vi "ReferenceMove Core.vi"(8 "error in (no error)":errorcluster, 10 "AxisNumber":u8, 11 "CS++Nanotec in":refnum<class "CS++Nanotec.lvclass">) -> (0 "error out":errorcluster, 3 "CS++Nanotec out":refnum<class "CS++Nanotec.lvclass">)   [LabVIEW 2015, in "CS++Nanotec.lvlib" / "CS++Nanotec.lvclass"]
doc: "Starts a movement to the reference switch of this axis. Once the motor reaches the reference switch it should slowly move down from the switch and stop. Afterwards the internal step counter is set to zero. \n\nThe main purpose of this function is to calibrate the motor."
uses:
  CS++Nanotec.lvclass
  CS++Nanotec.lvclass/CS++Nanotec.ctl
  instr.lib/NanotecSMCPD/NanotecSMCPDDriver.lvlib
  CSPP_DeviceBase/CS++Motor/CS++Motor.lvclass
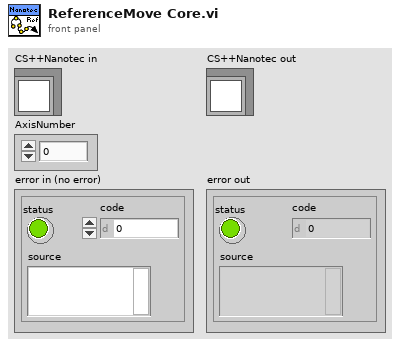
[diagram p1: front panel]
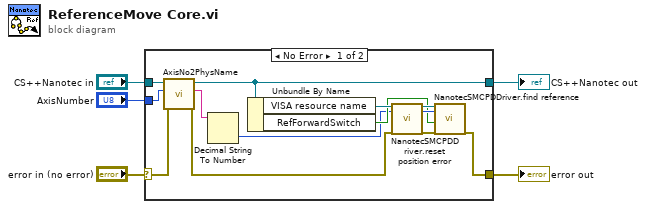
[diagram p0: block diagram]
diagram:
  n1 = case shown="No Error" "error in (no error)" {
    selector: "error in (no error)" -> [w9 w19]
    tunnel: "CS++Nanotec in" -> [w11 w20]
    tunnel: [w18 w19] -> w3
    tunnel: "AxisNumber" -> [w7 _]
    tunnel: [w10 w20] -> w1
    frame No Error {
      n2 = call "AxisNo2PhysName.vi"("error in (no error)"=w9, "AxisNumber"=w7, "CS++Motor in"=w11) -> ("error out"=w8:errorcluster, "PhysicalChannelName"=w12:string, "CS++Motor out"=w10:refnum<class "CS++Nanotec.lvclass">)  [unwired: 6 in]
      n3 = Decimal String To Number(string=w12) -> (number=w6:i32)  [unwired: 2 in, 1 out]
      n4 = Unbundle By Name(w10) -> ("VISA resource name"=w15:refnum<visa-resource-name>, "RefForwardSwitch"=w13:bool)
      n5 = call "NanotecSMCPDDriver.reset position error.vi"("VISA resource name"=w15, "contollerID"=w6, "error in (no error)"=w8) -> ("VISA resource name out"=w16:refnum<visa-resource-name>, "contollerID out"=w14:i32, "error out"=w17:errorcluster)  [unwired: 14 in]
      n6 = call "NanotecSMCPDDriver.find reference.vi"("VISA resource name"=w16, "contollerID"=w14, "forwardSwitch"=w13, "error in (no error)"=w17) -> ("error out"=w18:errorcluster)  [unwired: 13 in, 2 out]
    }
    frame Error {
    }
  }
  "error out" <- w3
  "CS++Nanotec out" <- w1
